vi "Main.vi"(11 "Module Admin":refnum<class "Delacor_lib_QMH_Module Admin.lvclass">) -> ()   [LabVIEW 2020, in "Panter Dashboard.lvlib"]
doc: "This template is based off of the Queued Message Handler design pattern and the Queued Message Handler project template that ships with LabVIEW.\n\nThe main difference is that the queue is private to this module and communication between modules is performed via Broadcast and Request events.\n\nRequest events are wrapped in public API methods and are handled in the Event Handling Loop (EHL) of this VI. Any module can register for Broadcast events sent by this module. The EHL generates messages based on user interface actions.\n\nThe Message Handling Loop (MHL) processes messages generated by the EHL, or by other messages. The messages are string values, so new messages can be added easily to the Message Cases case structure in the MHL. Each message cluster can also provide an optional value for Message Data, which is a variant that can be converted to whatever message-specific data is required.\n_____\nBased on DQMH Project Template 6.1.0.94."
uses:
  Panter Dashboard.lvlib
  <vilib>/Delacor/Delacor QMH/Libraries/Module Admin_class/Delacor_lib_QMH_Module Admin.lvclass
  Search button.ctl
  Module type--enum.ctl
  Module Data--cluster.ctl
  Maps List and refs--cluster.ctl
  <vilib>/National Instruments/Tree Map/Tree Map Data.ctl
  DQMH Modules Info--cluster.ctl
  Stop Argument--cluster.ctl
  <vilib>/Delacor/Delacor QMH/Libraries/Message Queue_class/Delacor_lib_QMH_Message Queue.lvclass/Delacor_lib_QMH_Message Queue.ctl
  Scan DQMH Modules Argument--cluster.ctl
  Tree DQMH Selection Argument--cluster.ctl
  Open Module API Tester Argument--cluster.ctl
  Open Event Front Panel Argument--cluster.ctl
  Execute Default Event Request Argument--cluster.ctl
  DQMH Tools Menu--enum.ctl
  Stop Module Instance Argument--cluster.ctl
  <vilib>/Delacor/Delacor QMH/Libraries/Module Admin_class/Delacor_lib_QMH_Module Admin.lvclass/Delacor_lib_QMH_Module Admin.ctl
  <vilib>/Delacor/Delacor QMH/Libraries/Module Admin_class/Delacor_lib_QMH_Get External Launch.vi
  <vilib>/Delacor/Delacor QMH/Libraries/Message Queue_class/Delacor_lib_QMH_Enqueue Message (Single).vi
  <vilib>/National Instruments/Tree Map/API/List Roots.vi
  <vilib>/National Instruments/Tree Map/Utility/Into Tree Control Items.vi
  <vilib>/Utility/error.llb/Error Cluster From Error Code.vi
  <vilib>/ErrorRing/Error Ring.xnode
  <vilib>/Delacor/Delacor QMH/Libraries/Message Queue_class/Delacor_lib_QMH_Message Queue.lvclass
  <vilib>/National Instruments/Tree Map/Tree Map.lvlib
panel:
  in  "Include Dependencies":bool
  in  "Scan Project For DQMH® Modules":T1
  in  "Modules Tree":string(tree) caption="Tree 2"
  out "Running?":bool
  out "Module type":T2
  out "Event Connector Pane":picture
  in  "Open Event FP":bool
  in  "Open API Tester":bool
  out "Module Description":string
  out "Event Description":string
  in  "Module ID":i32 caption="Numeric" format="Module ID : %d"
  in  "Show Diagram":bool
  in  "Hide Panel":bool
  in  "Show Panel":bool
  in  "Stop Instance":bool
  in  "Validate Module":bool
  in  "Rename Module":bool
  in  "Add Module":bool
  in  "Rename Event":bool
  in  "Convert Event":bool
  in  "Remove Event":bool
  in  "Add Event":bool
  out "Messages":string
  out "error out":errorcluster
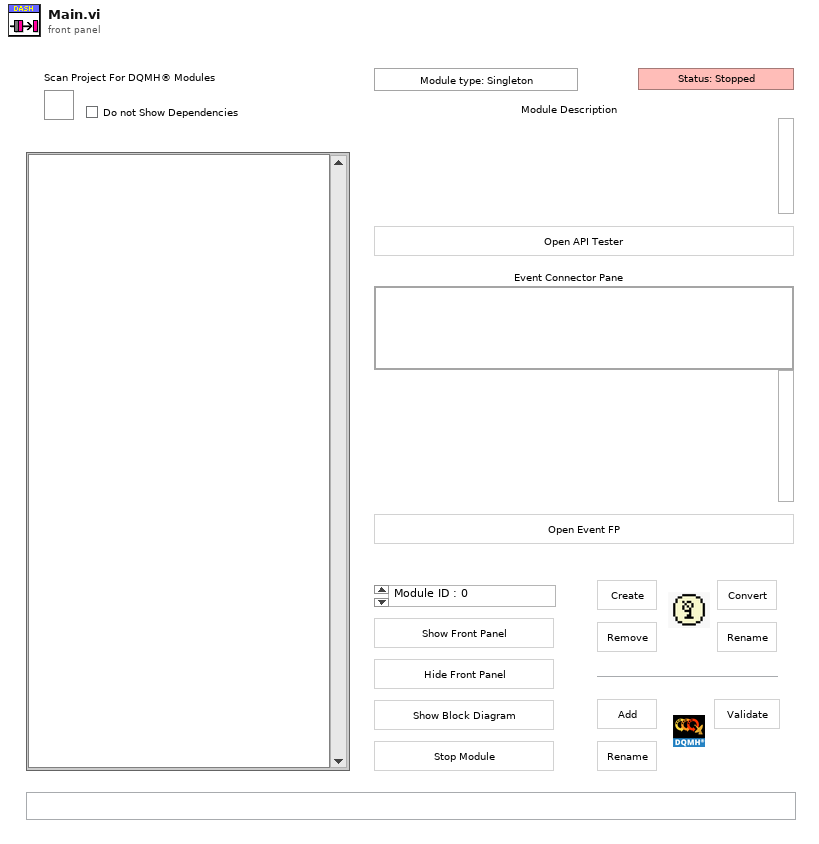
[diagram p1: front panel]
types:
  T1 = typedef "Panter Dashboard.lvlib/Search button.ctl" = bool
  T2 = typedef "Panter Dashboard.lvlib/Module type--enum.ctl" = enum16{"Module type: Singleton", "Module type: Cloneable"}
  T3 = typedef "Panter Dashboard.lvlib/Broadcast Events--cluster.ctl" = cluster{"Module Did Init":refnum<user-event>, "Status Updated":refnum<user-event>, "Error Reported":refnum<user-event>, "Module Did Stop":refnum<user-event>, "Update Module Execution Status":refnum<user-event>, "References Updated":refnum<user-event>}
  T4 = typedef "Panter Dashboard.lvlib/Request Events--cluster.ctl" = cluster{"Stop Module":refnum<user-event>, "Show Panel":refnum<user-event>, "Hide Panel":refnum<user-event>, "Get Module Execution Status":refnum<user-event>, "Show Diagram":refnum<user-event>, "Scan DQMH Modules":refnum<user-event>, "Tree DQMH Selection":refnum<user-event>, "Open Module API Tester":refnum<user-event>, "Open Event Front Panel":refnum<user-event>, "Execute Default Event Request":refnum<user-event>, "Stop Module Instance":refnum<user-event>}
  T5 = typedef "Panter Dashboard.lvlib/Module Data--cluster.ctl" = cluster{"DQMH Refs":cluster{"Event vi Ref":refnum<vi>, "DQMH Module Selected Ref":refnum<vi>}, "Status":string, "Maps":T6, "DQMH Modules Info":T8, "Module type":T2, "Module ID":i32}
  T6 = typedef "Panter Dashboard.lvlib/Maps List and refs--cluster.ctl" = cluster{"Tree Map":T7, "References Map":map{string, refnum<vi>}}
  T7 = typedef "Tree Map.lvlib/Tree Map Data.ctl" = map{string, cluster{"Child Paths Set":set{string}, "Name":string, "Data":string, "Attributes":map{string, string}}}
  T8 = typedef "Panter Dashboard.lvlib/DQMH Modules Info--cluster.ctl" = cluster{"DQMH Modules Refs":refnum<vi>[], "Modules List":string[], "Modules Descriptions":string[], "Modules Paths":path[], "Modules type":T2[]}
  T9 = enum32{"invalid lock state", "Not Locked", "Locked (No Password)", "Password-protected"}
  T10 = typedef "Panter Dashboard.lvlib/Stop Argument--cluster.ctl" = cluster{"Origin":string, "Exit via Stop Module Req?":bool, "Wait for Module to stop?":bool}
  T11 = typedef "Panter Dashboard.lvlib/Scan DQMH Modules Argument--cluster.ctl" = cluster{"Include Dependencies":bool}
  T12 = typedef "Panter Dashboard.lvlib/Tree DQMH Selection Argument--cluster.ctl" = cluster{"Tree DQMH Sel":string}
  T13 = typedef "Panter Dashboard.lvlib/Open Module API Tester Argument--cluster.ctl" = cluster{"Boolean":bool}
  T14 = typedef "Panter Dashboard.lvlib/Open Event Front Panel Argument--cluster.ctl" = cluster{"Boolean":bool}
  T15 = typedef "Panter Dashboard.lvlib/Execute Default Event Request Argument--cluster.ctl" = cluster{"Event Name":string}
  T16 = typedef "Panter Dashboard.lvlib/DQMH Tools Menu--enum.ctl" = enum16{"Create New DQMH Event", "Remove DQMH Event", "Convert DQMH Event", "Rename DQMH Event", "Add New DQMH Module", "Create RT Tester", "Rename DQMH Module", "Validate DQMH Module", "Create DQMH Module Template", "New DQMH  Unit Test"}
  T17 = typedef "Panter Dashboard.lvlib/Stop Module Instance Argument--cluster.ctl" = cluster{"Boolean":bool}
  T18 = enum32{"Invalid", "Standard", "Closed", "Hidden", "Minimized", "Maximized"}
  T19 = enum8{"Enabled", "Disabled", "Disabled and Grayed Out"}
  T20 = cluster{"Left Cell String":string, "Child Text":string[], "Child Tag":string, "Item Indent":i32, "Child Only?":bool, "Glyph Index":i32}[]
  T21 = typedef "Panter Dashboard.lvlib/Documentation--cluster.ctl" = cluster{"Module Description":string, "Event Description":string}
  T22 = cluster{"Vi out":refnum<vi>, "DQMH Lib":refnum<vi>}
  T23 = cluster{"Event vi Ref":refnum<vi>, "DQMH Module Selected Ref":refnum<vi>}
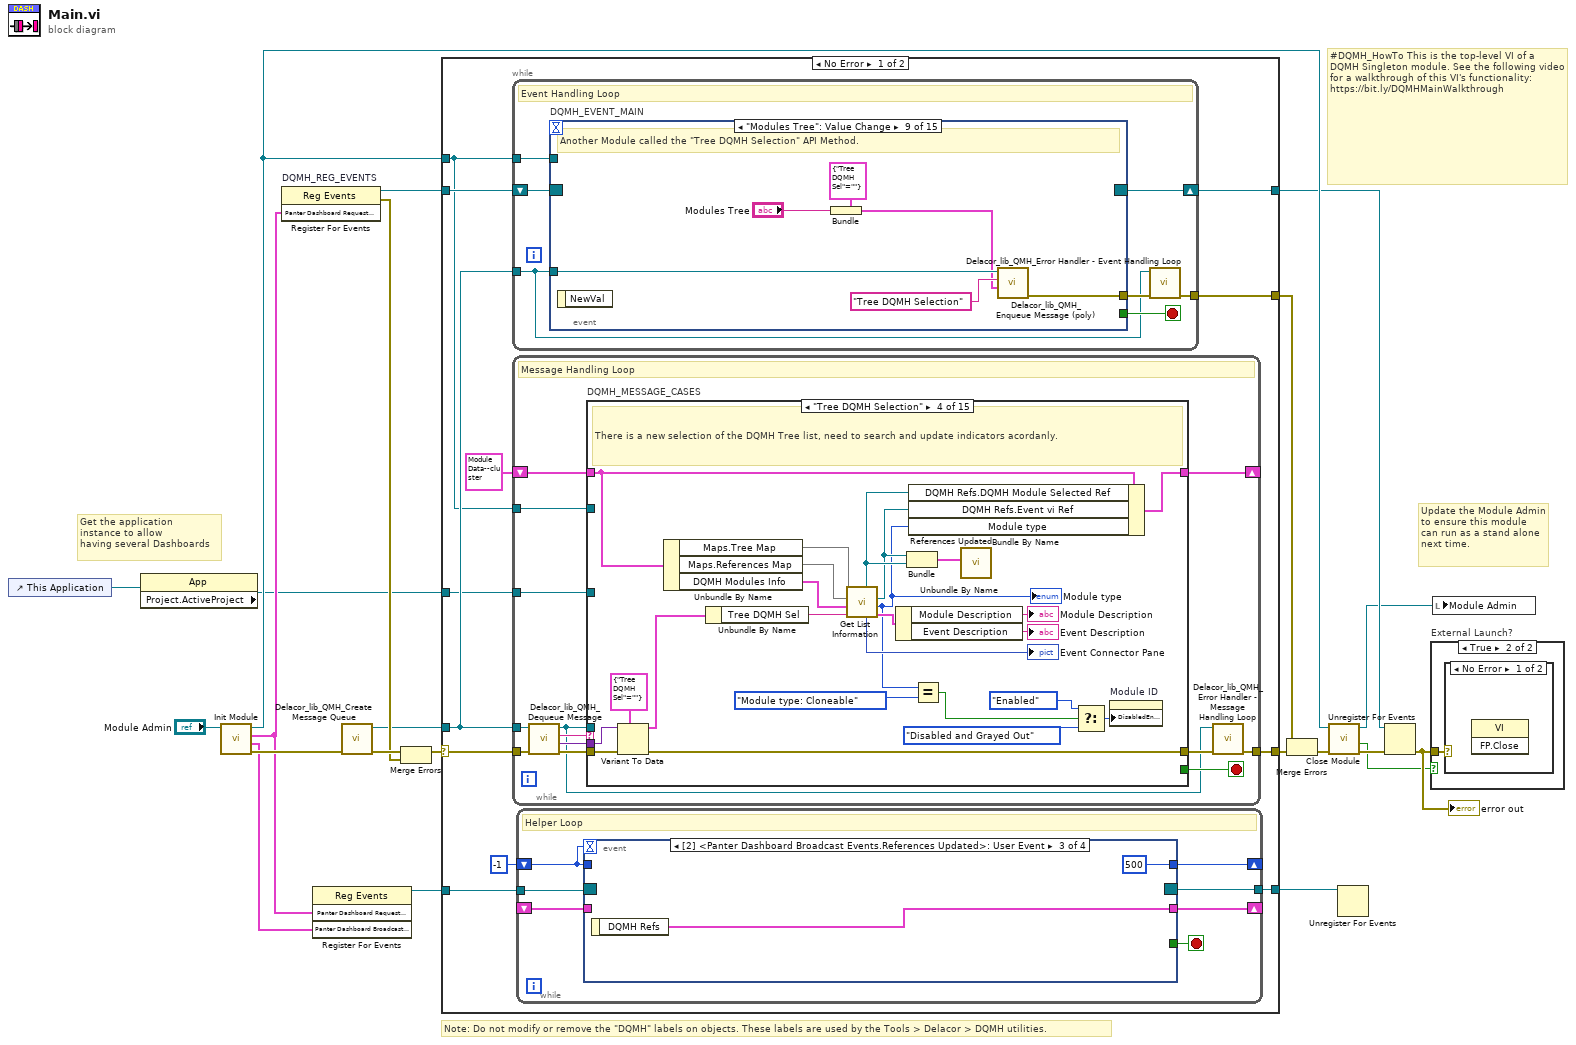
[diagram p0: block diagram]
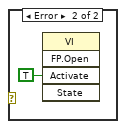
[diagram p3: hidden frame]
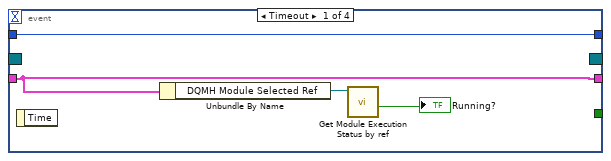
[diagram p4: hidden frame]
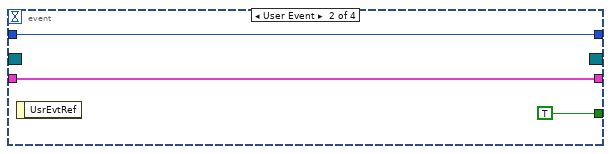
[diagram p5: hidden frame]
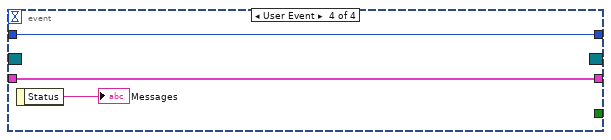
[diagram p6: hidden frame]
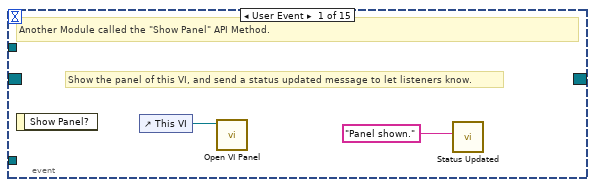
[diagram p7: hidden frame]
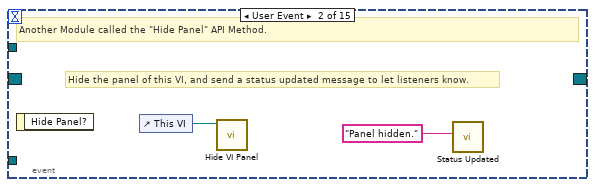
[diagram p8: hidden frame]
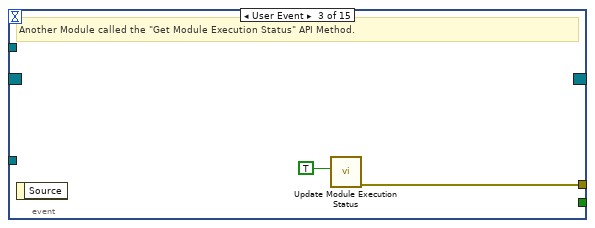
[diagram p9: hidden frame]
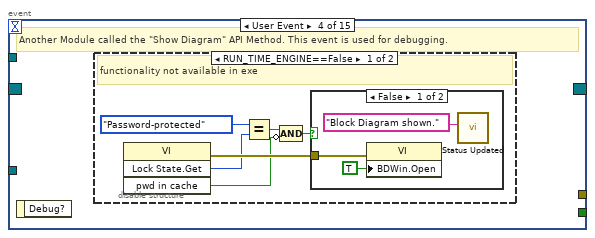
[diagram p10: hidden frame]
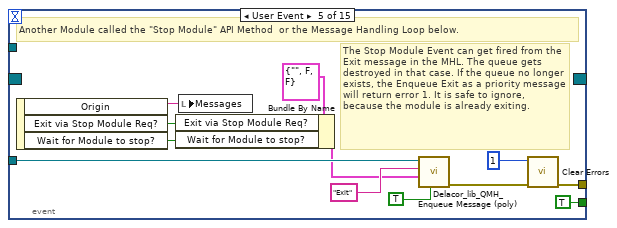
[diagram p13: hidden frame]
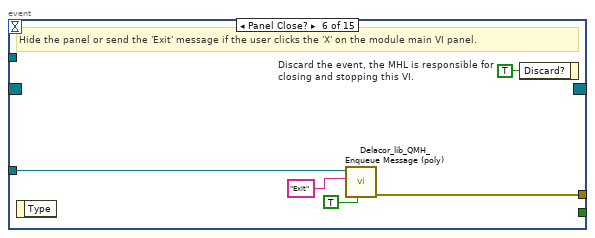
[diagram p14: hidden frame]
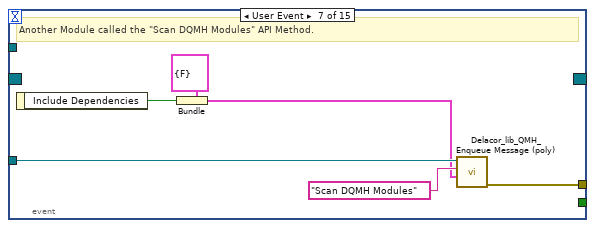
[diagram p15: hidden frame]
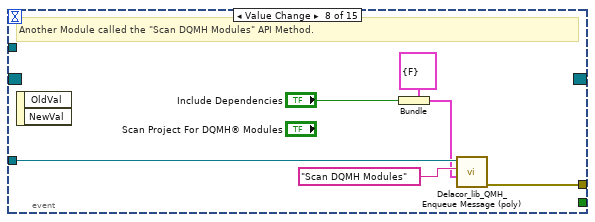
[diagram p16: hidden frame]
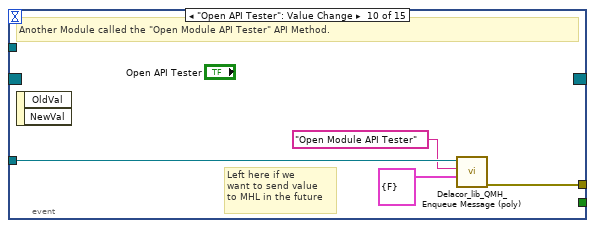
[diagram p17: hidden frame]
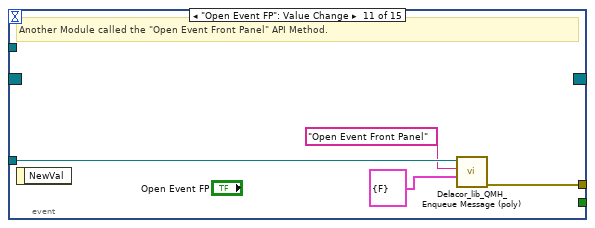
[diagram p18: hidden frame]
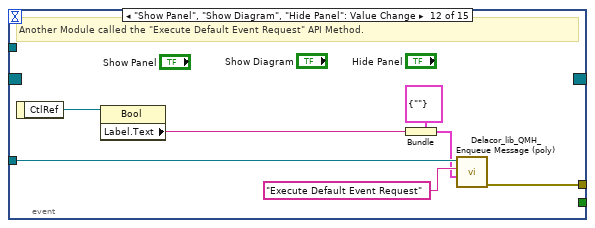
[diagram p19: hidden frame]
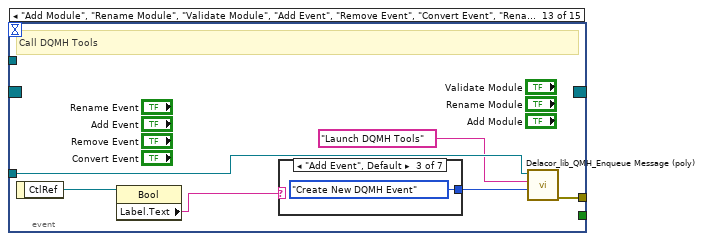
[diagram p20: hidden frame]
diagram:
  # "Get the application\ninstance to allow\nhaving several Dashboards"
  # "#DQMH_HowTo This is the top-level VI of a DQMH Singleton module. See the following video for a walkthrough of this VI's functionality: https://bit.ly/DQMHMainWalkthrough"
  # "Note: Do not modify or remove the \"DQMH\" labels on objects. These labels are used by the Tools > Delacor > DQMH utilities."
  # "Update the Module Admin to ensure this module can run as a stand alone next time."
  n1 = control-ref of="This Application"() -> (w2:refnum<vi>)
  n2 = property class="App"(reference=w2) -> ("Project.ActiveProject"=w1:refnum<vi>)  [unwired: 1 in, 2 out]
  n3 = call "Init Module.vi"("Singleton Module Admin in"="Module Admin") -> ("error out"=w21:errorcluster, "Panter Dashboard Broadcast Events"=w3:T3, "Panter Dashboard Request Events"=w4:T4, "Singleton Module Admin out"=w13:refnum<class "Delacor_lib_QMH_Module Admin.lvclass">)  [unwired: 7 in]
  n4 = register-events "DQMH_REG_EVENTS"(w4) -> (reference out=w11:refnum<event-registration>, error out=w14:errorcluster)  [unwired: 2 in]
  n5 = register-events(w4, w3) -> (reference out=w6:refnum<event-registration>)  [unwired: 2 in, 1 out]
  n6 = call <vilib>:"Delacor_lib_QMH_Create Message Queue.vi"("error in"=w21) -> ("error out"=w16:errorcluster, "Message Queue"=w10:refnum<class "Delacor_lib_QMH_Message Queue.lvclass">)  [unwired: 9 in]
  n7 = Merge Errors(w16, w14) -> (w15:errorcluster)
  n8 = case shown="No Error" w15 {
    selector: w15 -> [w32 w344]
    tunnel: [w34 w343] -> w22
    tunnel: [w31 w342] -> w12
    tunnel: w11 -> [w29 w342]
    tunnel: w10 -> [w28 w337]
    tunnel: [w33 _] -> w19
    tunnel: w13 -> [w27 w338]
    tunnel: w6 -> [w26 w336]
    tunnel: [w25 w336] -> w5
    tunnel: w1 -> [w23 _]
    frame No Error {
      n9 = while {
        tunnel: w28 -> [w54]
        shift-right: [w57] -> w31
        shift-left: w29 -> [w58]
        tunnel: [w59] -> w33
        tunnel: w27 -> [w55]
        stop <- w56 stop-if-true
        # "Event Handling Loop"
        n10 = event "DQMH_EVENT_MAIN" shown="[8] \"Modules Tree\": Value Change" {
          selector: w58 -> [_ _ _ _ _ _ _ _ _ _ _ _ _ _ _]
          dyn-events: [_ _ _ _ _ _ _ _ _ _ _ _ _ _ _] -> w57
          timeout: _ -> [_ _ _ _ _ _ _ _ _ _ _ _ _ _ _]
          tunnel: [_ _ _ _ TRUE ("Discard?") _ _ _ _ _ _ _ _ _ _] -> w56
          tunnel: w54 -> [_ _ _ _ w83 w90 w97 w103 w109 w113 w117 w124 w130 w141 w145]
          tunnel: [_ _ w66 _ w86 w92 w98 w104 w110 w114 w118 w125 w131 w142 w146] -> w60
          tunnel: w55 -> [_ _ _ _ _ _ _ _ _ _ _ _ _ _ _]
          event User Event {
            # "Show the panel of this VI, and send a status updated message to let listeners know."
            # "Another Module called the \"Show Panel\" API Method."
            n11 = event-data() -> ()  [unwired: 1 in, 1 out]
            n12 = control-ref of="This VI"() -> (w62:refnum<vi>)
            n13 = call "Open VI Panel.vi"("VI"=w62) -> ()  [unwired: 10 in, 1 out]
            n14 = call "Status Updated.vi"("Status"="Panel shown." ("format string")) -> ()  [unwired: 10 in, 1 out]
          }
          event User Event {
            # "Hide the panel of this VI, and send a status updated message to let listeners know."
            # "Another Module called the \"Hide Panel\" API Method."
            n15 = event-data() -> ()  [unwired: 1 in, 1 out]
            n16 = control-ref of="This VI"() -> (w64:refnum<vi>)
            n17 = call "Hide VI Panel.vi"("VI"=w64) -> ()  [unwired: 10 in, 1 out]
            n18 = call "Status Updated.vi"("Status"="Panel hidden." ("format string")) -> ()  [unwired: 10 in, 1 out]
          }
          event User Event {
            # "Another Module called the \"Get Module Execution Status\" API Method."
            n19 = event-data() -> ()  [unwired: 1 in, 1 out]
            n20 = call "Update Module Execution Status.vi"("Running?"=TRUE) -> ("error out"=w66:errorcluster)  [unwired: 10 in]
          }
          event User Event {
            # "Another Module called the \"Show Diagram\" API Method. This event is used for debugging."
            n21 = event-data() -> ()  [unwired: 1 in, 1 out]
            n22 = disable-structure shown="RUN_TIME_ENGINE==False" {
              frame condition #0 (active) {
                # "functionality not available in exe"
                n23 = invoke class="VI" method="Lock State.Get"() -> (error out=w72:errorcluster, "Get Lock State"=w71:T9, "pwd in cache"=w68:bool)  [unwired: 4 in, 1 out]
                n24 = Equal?(x=T9."Password-protected", y=w71) -> (x = y?=w69:bool)
                n25 = Compound Arithmetic op=AND(w69, invert w68) -> (w67:bool)
                n26 = case shown="False" w67 {
                  tunnel: w72 -> [w75 _]
                  frame False {
                    n27 = property class="VI"(error in=w75, "BDWin.Open"=TRUE ("Block Diagram Window:Open")) -> ()  [unwired: 1 in, 2 out]
                    n28 = call "Status Updated.vi"("Status"="Block Diagram shown." ("format string")) -> ()  [unwired: 10 in, 1 out]
                  }
                  frame True {
                    # "Password-protected VI, and the password is not in the cache. Do not show the diagram."
                  }
                }
              }
              frame condition #1 {
              }
            }
          }
          event User Event {
            # "The Stop Module Event can get fired from the Exit message in the MHL. The queue gets destroyed in that case. If the queue no longer exists, the Enqueue Exit as a priority message will return error 1. It is safe to ignore, because the module is already exiting."
            # "Another Module called the \"Stop Module\" API Method  or the Message Handling Loop below."
            n29 = event-data() -> ("Origin"=w82:string, "Exit via Stop Module Req?"=w78:bool, "Wait for Module to stop?"=w77:bool)  [unwired: 1 in]
            n30 = Bundle By Name(cluster=T10 {"Origin"="", "Exit via Stop Module Req?"=FALSE, "Wait for Module to stop?"=FALSE} ("Stop Argument"), "Exit via Stop Module Req?"=w78, "Wait for Module to stop?"=w77) -> (w76:T10)
            n31 = local write "Messages"(w82) -> ()
            n32 = call-poly <vilib>:"Delacor_lib_QMH_Enqueue Message (poly).vi"("Priority Message? (F)"=TRUE, "Message Data"=w76, "Message"="Exit", "Message Queue in"=w83) -> ("error out"=w87:errorcluster)  [unwired: 6 in, 1 out]
            n33 = call <vilib>:"Clear Errors.vi"("error in (no error)"=w87, "specific error code to clear (0: all)"=1) -> ("error out"=w86:errorcluster)  [unwired: 4 in, 1 out]
          }
          event Panel Close? {
            w91 = TRUE  # Discard the event, the MHL is responsible for closing and stopping this VI.
            # "Hide the panel or send the 'Exit' message if the user clicks the 'X' on the module main VI panel."
            n34 = event-data() -> ()  [unwired: 1 in, 1 out]
            n35 = call-poly <vilib>:"Delacor_lib_QMH_Enqueue Message (poly).vi"("Priority Message? (F)"=TRUE, "Message"="Exit", "Message Queue in"=w90) -> ("error out"=w92:errorcluster)  [unwired: 7 in, 1 out]
            n36 = event-data("Discard?"=w91) -> ()  [unwired: 1 in, 1 out]
          }
          event User Event {
            # "Another Module called the \"Scan DQMH Modules\" API Method."
            n37 = event-data() -> ("Include Dependencies"=w93:bool)  [unwired: 1 in]
            n38 = Bundle(cluster=T11 {"Include Dependencies"=FALSE} ("Scan DQMH Modules Argument"), "Include Dependencies"=w93) -> (w94:T11)
            n39 = call-poly <vilib>:"Delacor_lib_QMH_Enqueue Message (poly).vi"("Message Data"=w94, "Message"="Scan DQMH Modules", "Message Queue in"=w97) -> ("error out"=w98:errorcluster)  [unwired: 7 in, 1 out]
          }
          event Value Change {
            # "Another Module called the \"Scan DQMH Modules\" API Method."
            n40 = event-data() -> ()  [unwired: 1 in, 2 out]
            n41 = Bundle(cluster=T11 {"Include Dependencies"=FALSE} ("Scan DQMH Modules Argument"), "Include Dependencies"="Include Dependencies") -> (w100:T11)
            n42 = call-poly <vilib>:"Delacor_lib_QMH_Enqueue Message (poly).vi"("Message Data"=w100, "Message"="Scan DQMH Modules", "Message Queue in"=w103) -> ("error out"=w104:errorcluster)  [unwired: 7 in, 1 out]
          }
          event "Modules Tree": Value Change {
            # "Another Module called the \"Tree DQMH Selection\" API Method."
            n43 = event-data() -> ()  [unwired: 1 in, 1 out]
            n44 = Bundle(cluster=T12 {"Tree DQMH Sel"=""} ("Tree DQMH Selection Argument"), "Tree DQMH Sel"="Modules Tree") -> (w106:T12)
            n45 = call-poly <vilib>:"Delacor_lib_QMH_Enqueue Message (poly).vi"("Message Data"=w106, "Message"="Tree DQMH Selection", "Message Queue in"=w109) -> ("error out"=w110:errorcluster)  [unwired: 7 in, 1 out]
          }
          event "Open API Tester": Value Change {
            # "Left here if we\nwant to send value\nto MHL in the future"
            # "Another Module called the \"Open Module API Tester\" API Method."
            n46 = event-data() -> ()  [unwired: 1 in, 2 out]
            n47 = call-poly <vilib>:"Delacor_lib_QMH_Enqueue Message (poly).vi"("Message Data"=T13 {"Boolean"=FALSE} ("Open Module API Tester Argument"), "Message"="Open Module API Tester", "Message Queue in"=w113) -> ("error out"=w114:errorcluster)  [unwired: 7 in, 1 out]
          }
          event "Open Event FP": Value Change {
            # "Another Module called the \"Open Event Front Panel\" API Method."
            n48 = event-data() -> ()  [unwired: 1 in, 1 out]
            n49 = call-poly <vilib>:"Delacor_lib_QMH_Enqueue Message (poly).vi"("Message Data"=T14 {"Boolean"=FALSE} ("Open Event Front Panel Argument"), "Message"="Open Event Front Panel", "Message Queue in"=w117) -> ("error out"=w118:errorcluster)  [unwired: 7 in, 1 out]
          }
          event "Show Panel", "Show Diagram", "Hide Panel": Value Change {
            # "Another Module called the \"Execute Default Event Request\" API Method."
            n50 = event-data() -> ("CtlRef"=w120:refnum<vi>)  [unwired: 1 in]
            n51 = property class="Bool"(reference=w120) -> ("Label.Text"=w119:string)  [unwired: 1 in, 2 out]
            n52 = Bundle(cluster=T15 {"Event Name"=""} ("Execute Default Event Request Argument"), "Event Name"=w119) -> (w121:T15)
            n53 = call-poly <vilib>:"Delacor_lib_QMH_Enqueue Message (poly).vi"("Message Data"=w121, "Message"="Execute Default Event Request", "Message Queue in"=w124) -> ("error out"=w125:errorcluster)  [unwired: 7 in, 1 out]
          }
          event "Add Module", "Rename Module", "Validate Module", "Add Event", "Remove Event", "Convert Event", "Rename Event": Value Change {
            # "Call DQMH Tools"
            n54 = event-data() -> ("CtlRef"=w127:refnum<vi>)  [unwired: 1 in]
            n55 = property class="Bool"(reference=w127) -> ("Label.Text"=w126:string)  [unwired: 1 in, 2 out]
            n56 = case shown="\"Add Event\", Default" w126 {
              tunnel: [DQMH_Tools_Menu--enum."Remove DQMH Event" ("DQMH Tools") DQMH_Tools_Menu--enum."Rename DQMH Event" ("DQMH Tools") DQMH_Tools_Menu--enum."Create New DQMH Event" ("DQMH Tools") DQMH_Tools_Menu--enum."Convert DQMH Event" ("DQMH Tools") DQMH_Tools_Menu--enum."Add New DQMH Module" ("DQMH Tools") DQMH_Tools_Menu--enum."Validate DQMH Module" ("DQMH Tools") DQMH_Tools_Menu--enum."Rename DQMH Module" ("DQMH Tools")] -> w128
              frame "Remove Event" {
              }
              frame "Rename Event" {
              }
              frame "Add Event", Default {
              }
              frame "Convert Event" {
              }
              frame "Add Module" {
              }
              frame "Validate Module" {
              }
              frame "Rename Module" {
              }
            }
            n57 = call-poly <vilib>:"Delacor_lib_QMH_Enqueue Message (poly).vi"("Message Data"=w128, "Message"="Launch DQMH Tools", "Message Queue in"=w130) -> ("error out"=w131:errorcluster)  [unwired: 7 in, 1 out]
          }
          event "Stop Instance": Value Change {
            # "Another Module called the \"Stop Module Instance\" API Method."
            n58 = event-data() -> ()  [unwired: 1 in, 1 out]
            n59 = call-poly <vilib>:"Delacor_lib_QMH_Enqueue Message (poly).vi"("Message Data"=T17 {"Boolean"=FALSE} ("Stop Module Instance Argument"), "Message"="Stop Module Instance", "Message Queue in"=w141) -> ("error out"=w142:errorcluster)  [unwired: 7 in, 1 out]
          }
          event "Module ID": Value Change {
            # "Module ID has value change"
            n60 = event-data() -> ()  [unwired: 1 in, 1 out]
            n61 = call-poly <vilib>:"Delacor_lib_QMH_Enqueue Message (poly).vi"("Message Data"="Module ID", "Message"="Module ID Update", "Message Queue in"=w145) -> ("error out"=w146:errorcluster)  [unwired: 7 in, 1 out]
          }
        }
        n62 = call-dynamic "Delacor_lib_QMH_Error Handler - Event Handling Loop.vi"("error in"=w60, "Message Queue in"=w54) -> ("dup error in"=w59:errorcluster)  [unwired: 8 in, 1 out]
      }
      n63 = while {
        tunnel: w28 -> [w150]
        shift-right: [w154] -> _
        shift-left: T5 {"DQMH Refs"={"Event vi Ref"=refnum, "DQMH Module Selected Ref"=refnum}, "Status"="", "Maps"={"Tree Map"={}, "References Map"={}}, "DQMH Modules Info"={"DQMH Modules Refs"=[], "Modules List"=[], "Modules Descriptions"=[], "Modules Paths"=[], "Modules type"=[]}, "Module type"=enum."Module type: Singleton", "Module ID"=0} ("Data Cluster") -> [w155]
        tunnel: w32 -> [w158]
        tunnel: [w156] -> w34
        tunnel: w27 -> [w148]
        tunnel: w23 -> [w147]
        stop <- w153 stop-if-true
        # "Message Handling Loop"
        n64 = call-dynamic "Delacor_lib_QMH_Dequeue Message.vi"("error in"=w158, "Message Queue in"=w150) -> ("error out"=w157:errorcluster, "Message Data"=w151:variant, "Message"=w152:string, "Message Queue out"=w149:refnum<class "Delacor_lib_QMH_Message Queue.lvclass">)  [unwired: 6 in]
        n65 = case "DQMH_MESSAGE_CASES" shown="\"Tree DQMH Selection\"" w152 {
          selector: w152 -> [_ _ _ _ _ _ _ _ _ _ _ _ _ _ w323]
          tunnel: w149 -> [_ _ _ _ _ _ _ _ _ _ _ _ w292 w315 _]
          tunnel: w157 -> [w180 w184 w202 w226 w233 w242 w253 w266 w277 w284 w287 w289 w299 w321 w325]
          tunnel: [w178 w184 w200 w225 w232 w241 w252 w264 w275 w283 w286 w289 w295 w318 w326] -> w159
          tunnel: w155 -> [w169 w183 w185 w220 w230 w238 w247 w259 w271 w282 w285 w288 w294 w307 w324]
          tunnel: [w168 w183 w195 w212 w230 w238 w247 w259 w271 w280 w285 w288 w294 w307 w324] -> w154
          tunnel: [_ _ _ _ _ _ _ _ _ _ _ _ _ w314 _] -> w153
          tunnel: w151 -> [_ _ w198 w224 w229 w240 w251 w262 w273 w281 _ _ w293 w313 _]
          tunnel: w148 -> [w170 _ _ _ _ _ _ _ _ _ _ _ w291 w308 _]
          tunnel: w147 -> [w163 _ w187 _ _ _ _ _ _ _ _ _ _ _ _]
          frame "Initialize" {
            w164 = "Panther Dash " ("Initial Message")
            # "Initialize - Any operation that needs to be done before the module can receive messages. Synchronize Caller Events.vi will inform Start Module.vi that the module has launched and is ready to receive messages. Module Did Init.vi will broadcast that the module initialized."
            n66 = call "Synchronize Caller Events.vi"("error in (no error)"=w180, "Singleton Module Admin in"=w170) -> ("error out"=w179:errorcluster, "Singleton Module Admin out"=w165:refnum<class "Delacor_lib_QMH_Module Admin.lvclass">)  [unwired: 8 in]
            n67 = property class="Project"(reference=w163) -> ("Name"=w162:string)  [unwired: 1 in, 2 out]
            n68 = property class="Module Admin"(reference=w165) -> ("Accessors:External Launch"=w174:bool)  [unwired: 1 in, 2 out]
            n69 = invoke on="Modules Tree" class="Tree (strict)" method="Edit Tree Items.Delete"() -> ()  [unwired: 5 in, 5 out]
            n70 = Select(t=T18."Hidden" ("State"), s=w174, f=T18."Standard" ("State")) -> (s? t:f=w171:T18)
            n71 = Format Into String(format string="Panther Dasboard for DQMH® : %s", w162) -> (resulting string=w161:string, error out=w177:errorcluster)  [unwired: 2 in]
            n72 = property class="VI"(error in=w177, "Front Panel.Title"=w161) -> (reference out=w176:refnum<vi>, error out=w182:errorcluster)  [unwired: 1 in]
            n73 = call "Module Name--constant.vi"() -> ("Module Name"=w166:string)  [unwired: 11 in]
            n74 = invoke class="VI" method="FP.Open"(reference=w176, error in=w182, "State"=w171) -> (reference out=w175:refnum<vi>, error out=w181:errorcluster)  [unwired: 2 in, 3 out]
            n75 = Bundle By Name(cluster=w169, "Status"=w164) -> (w168:T5)
            n76 = local write "Messages"(w164) -> ()
            n77 = call "Module Did Init.vi"("error in (no error)"=w179, "Initialized?"=TRUE, "Origin"=w166) -> ("error out"=w178:errorcluster)  [unwired: 8 in]
            n78 = invoke class="VI" method="FP.Center"(reference=w175, error in=w181) -> ()  [unwired: 1 in, 3 out]
          }
          frame "---Module Specific---" {
            # "Separator -- The following cases handle messages specific to this Module."
          }
          frame "Scan DQMH Modules" {
            # "Scan DQMH Modules in the project and fill 2 maps one with the Vi References and the another one with the list of DQMH modules on the project"
            n79 = Variant To Data(error in=w202, type=T11 {"Include Dependencies"=FALSE} ("Scan DQMH Modules Argument"), Variant=w198) -> (data=w196:T11, error out=w201:errorcluster)
            n80 = Unbundle By Name(w196) -> ("Include Dependencies"=w186:bool)
            n81 = local write "Include Dependencies"(w186) -> ()
            n82 = call "Get Panther Dash Library.vi"() -> ("Library out"=w193:refnum<vi>)  [unwired: 11 in]
            n83 = call "Scan DQMH Modules and create Maps.vi"("Panther Dash DQMH Lib"=w193, "Include Dependencies"=w186, "Project"=w187) -> ("error out"=w199:errorcluster, "Tree Map out"=w188:T7, "map ref out"=w189:map{string, refnum<vi>}, "DQMH Modules Info"=w194:T8)  [unwired: 5 in]
            n84 = control-ref of="Modules Tree"() -> (w190:refnum<vi>)
            n85 = Bundle By Name(cluster=w185, "DQMH Modules Info"=w194, "Maps.References Map"=w189, "Maps.Tree Map"=w188) -> (w195:T5)
            n86 = call <vilib>:"Tree Map to Tree Control Items.vi"("Tree Map In"=w188) -> ("Tree Control Items"=w191:T20)  [unwired: 10 in]
            n87 = call "Draw Tree.vi"("Tree Control Items"=w191, "TreeControl in"=w190) -> ()  [unwired: 9 in, 1 out]
            n88 = Merge Errors(w201, w199) -> (w200:errorcluster)
            n89 = call "Status Updated.vi"("Status"="Scanning DQMH Modules") -> ()  [unwired: 10 in, 1 out]
          }
          frame "Tree DQMH Selection" {
            # "There is a new selection of the DQMH Tree list, need to search and update indicators acordanly."
            n90 = Variant To Data(error in=w226, type=T12 {"Tree DQMH Sel"=""} ("Tree DQMH Selection Argument"), Variant=w224) -> (data=w222:T12, error out=w225:errorcluster)
            n91 = Unbundle By Name(w220) -> ("Maps.Tree Map"=w219:T7, "Maps.References Map"=w218:map{string, refnum<vi>}, "DQMH Modules Info"=w217:T8)
            n92 = Unbundle By Name(w222) -> ("Tree DQMH Sel"=w221:string)
            n93 = call "Get List Information.vi"("List Selection"=w221, "DQMH Modules Info"=w217, "References Map"=w218, "Tree Map"=w219) -> ("Documentation"=w215:T21, "Module Type"=w205:T2, "Vi out"=w210:refnum<vi>, "VI Connector Pane"=→"Event Connector Pane":picture, "DQMH Lib"=w211:refnum<vi>)  [unwired: 2 in, 1 out]
            "Module type" <- w205
            n94 = Unbundle By Name(w215) -> ("Module Description"=→"Module Description":string, "Event Description"=→"Event Description":string)
            n95 = Bundle("Vi out"=w210, "DQMH Lib"=w211) -> (w209:T22)  [unwired: 1 in]
            n96 = Bundle By Name(cluster=w220, "DQMH Refs.DQMH Module Selected Ref"=w211, "DQMH Refs.Event vi Ref"=w210, "Module type"=w205) -> (w212:T5)
            n97 = Equal?(x=w205, y=Module_type--enum."Module type: Cloneable") -> (x = y?=w204:bool)
            n98 = call "References Updated.vi"("DQMH Refs"=w209) -> ()  [unwired: 10 in, 1 out]
            n99 = Select(t=T19."Enabled" ("Disabled"), s=w204, f=T19."Disabled and Grayed Out") -> (s? t:f=w207:T19)
            n100 = property on="Module ID" class="DigNum (strict)"("DisabledEnum"=w207) -> ()  [unwired: 2 in, 2 out]
          }
          frame "Launch DQMH Tools" {
            # "Launch DQMH Tools"
            n101 = Variant To Data(error in=w233, type=DQMH_Tools_Menu--enum."Create New DQMH Event" ("DQMH Tools"), Variant=w229) -> (data=w227:T16, error out=w231:errorcluster)
            n102 = call "Launch DQMH Tools by menu.vi"("error in"=w231, "DQMH Tools"=w227) -> ("error out"=w232:errorcluster)  [unwired: 9 in]
          }
          frame "Open Module API Tester" {
            # "Open the API Tester from the selected DQMH Module"
            n103 = Variant To Data(error in=w242, type=T13 {"Boolean"=FALSE} ("Open Module API Tester Argument"), Variant=w240) -> ()  [unwired: 2 out]
            n104 = Unbundle By Name(w238) -> ("DQMH Refs.DQMH Module Selected Ref"=w236:refnum<vi>)
            n105 = property class="Library"(reference=w236) -> ("Name"=w235:string)  [unwired: 1 in, 2 out]
            n106 = call "Open API Tester.vi"("DQMH Library Ref"=w236) -> ("error out"=w241:errorcluster)  [unwired: 10 in]
            n107 = Format Into String(format string="Open: %s  API Tester " ("Status"), w235) -> (resulting string=w234:string)  [unwired: 2 in, 1 out]
            n108 = call "Status Updated.vi"("Status"=w234) -> ()  [unwired: 10 in, 1 out]
          }
          frame "Open Event Front Panel" {
            # "Open the Front Panel from the selected Event from the tree"
            n109 = Variant To Data(error in=w253, type=T14 {"Boolean"=FALSE} ("Open Event Front Panel Argument"), Variant=w251) -> ()  [unwired: 2 out]
            n110 = Unbundle By Name(w247) -> ("DQMH Refs.Event vi Ref"=w246:refnum<vi>)
            n111 = invoke class="VI" method="FP.Open"(reference=w246, "Activate"=TRUE ("Wait Until Done"), "State"=T18."Standard") -> (error out=w252:errorcluster)  [unwired: 2 in, 4 out]
            n112 = property class="VI"(reference=w246) -> ("Name"=w245:string)  [unwired: 1 in, 2 out]
            n113 = Format Into String(format string="Front Panel : %s Opened", w245) -> (resulting string=w244:string)  [unwired: 2 in, 1 out]
            n114 = call "Status Updated.vi"("Status"=w244) -> ()  [unwired: 10 in, 1 out]
          }
          frame "Execute Default Event Request" {
            # "Execute Default Event"
            n115 = Unbundle By Name(w259) -> ("Maps.References Map"=w258:map{string, refnum<vi>}, "DQMH Refs.DQMH Module Selected Ref"=w257:refnum<vi>, "Module type"=w255:T2, "Module ID"=w254:i32)
            n116 = Variant To Data(error in=w266, type=T15 {"Event Name"=""} ("Execute Default Event Request Argument"), Variant=w262) -> (data=w260:T15, error out=w265:errorcluster)
            n117 = Unbundle By Name(w260) -> ("Event Name"=w256:string)
            n118 = call "Execute default event by ID.vi"("Event Name"=w256, "Module ID"=w254, "Module type"=w255, "Module Lib"=w257, "References Map"=w258) -> ("error out"=w263:errorcluster)  [unwired: 6 in]
            n119 = Merge Errors(w265, w263) -> (w264:errorcluster)
          }
          frame "Stop Module Instance" {
            # "Execute the Stop Module Request, when Cloneable type this Request uses the Module ID"
            n120 = Variant To Data(error in=w277, type=T17 {"Boolean"=FALSE} ("Stop Module Instance Argument"), Variant=w273) -> (error out=w276:errorcluster)  [unwired: 1 out]
            n121 = Unbundle By Name(w271) -> ("Maps.References Map"=w270:map{string, refnum<vi>}, "DQMH Refs.DQMH Module Selected Ref"=w269:refnum<vi>, "Module type"=w268:T2, "Module ID"=w267:i32)
            n122 = call "Stop DQMH Module.vi"("Module ID"=w267, "Module type"=w268, "Module Lib"=w269, "References Map"=w270) -> ("error out"=w274:errorcluster)  [unwired: 7 in]
            n123 = Merge Errors(w276, w274) -> (w275:errorcluster)
          }
          frame "Module ID Update" {
            # "Module ID Control has value change"
            n124 = Variant To Data(error in=w284, type=0 ("Module ID"), Variant=w281) -> (data=w279:i32, error out=w283:errorcluster)
            n125 = Bundle By Name(cluster=w282, "Module ID"=w279) -> (w280:T5)
          }
          frame "---Copy This Frame---" {
            # "Duplicate this frame when creating new messages.  Change this comment in the duplicated frame to describe this message."
            n126 = Merge Errors(w287) -> (w286:errorcluster)
          }
          frame "---Exit and Error Handling---" {
            # "Separator - The following cases handle errors and exit messages."
          }
          frame "Error" {
            # "#CodeRecommended - If you ever change the name of this \"Error\" message, you'll need to update the name in the Check Loop Error.vi as well."
            # "#CodeRecommended - If the module is running in standalone mode (External Launch = FALSE), this code will pop up an error dialog and call the 'Exit' message if an error occurs. Add more fine-grained error handling here."
            # "Error - Check the error message data and respond accordingly. This message is sent by the \"Error Handler\" VIs at the end of each loop in this application."
            n127 = property class="Module Admin"(reference=w291) -> ("Accessors:External Launch"=w290:bool)  [unwired: 1 in, 2 out]
            n128 = Variant To Data(error in=w299, type=errorcluster {"status"=FALSE, "code"=0, "source"=""} ("error constant"), Variant=w293) -> (data=w300:errorcluster, error out=w297:errorcluster)
            n129 = call "Error Reported.vi"("Error"=w300) -> ()  [unwired: 10 in, 1 out]
            n130 = case shown="False" w290 {
              tunnel: [w305 _] -> w296
              tunnel: w292 -> [w303 _]
              tunnel: w300 -> [w304 _]
              frame False {
                # "If the module is running standalone, then pop up an error dialog and call the \"Exit\" message."
                n131 = call <vilib>:"Simple Error Handler.vi"("error in (no error)"=w304) -> ()  [unwired: 4 in, 5 out]
                n132 = call-poly <vilib>:"Delacor_lib_QMH_Enqueue Message (poly).vi"("Priority Message? (F)"=TRUE, "Message"="Exit", "Message Queue in"=w303) -> ("error out"=w305:errorcluster)  [unwired: 7 in, 1 out]
              }
              frame True {
                # "If the module was launched externally, calling the Error Reported broadcast VI is the only action performed by the \"Error\" message. The module's caller can then process the error appropriately."
              }
            }
            n133 = Merge Errors(w297, w296) -> (w295:errorcluster)
            n134 = local write "error out"(w295) -> ()
          }
          frame "Exit" {
            w312 = 91  # 91: not all Exit messages will have an argument
            w314 = TRUE  # Stop the VI
            # "Release the message queue reference"
            # "#CodeNeeded - Add any required cleanup code here"
            # "Exit - Exit the application."
            n135 = Variant To Data(error in=w321, type=T10 {"Origin"="", "Exit via Stop Module Req?"=FALSE, "Wait for Module to stop?"=FALSE} ("Stop Argument"), Variant=w313) -> (data=w310:T10, error out=w317:errorcluster)
            n136 = call <vilib>:"Clear Errors.vi"("error in (no error)"=w317, "specific error code to clear (0: all)"=w312) -> ("error out"=w320:errorcluster)  [unwired: 4 in, 1 out]
            n137 = control-ref of="This VI"() -> (w309:refnum<vi>)
            n138 = call-dynamic "Delacor_lib_QMH_Release Message Queue.vi"("error in"=w320, "Message Queue"=w315) -> ("error out"=w319:errorcluster)  [unwired: 9 in]
            n139 = call "Handle Exit.vi"("Stop Argument"=w310, "Admin in"=w308, "VI reference"=w309) -> ("error out"=w316:errorcluster)  [unwired: 7 in, 1 out]
            n140 = Unbundle By Name(w307) -> ("Maps.References Map"=w306:map{string, refnum<vi>})
            n141 = Merge Errors(w319, w316) -> (w318:errorcluster)
            n142 = call "Close vi references.vi"("map"=w306) -> ()  [unwired: 10 in, 1 out]
          }
          frame Default {
            # "'Default' case only runs if there is a message that isn't defined in any of the other cases.  Output a programming error."
            n143 = call "Module Name--constant.vi"() -> ("Module Name"=w322:string)  [unwired: 11 in]
            n144 = xnode "Error Ring"("parameter 0"=w323, "parameter 1"=w322) -> ("error out"=w327:errorcluster)
            n145 = Merge Errors(w325, w327) -> (w326:errorcluster)
          }
        }
        n146 = call-dynamic "Delacor_lib_QMH_Error Handler - Message Handling Loop.vi"("error in"=w159, "Message Queue in"=w149) -> ("dup error in"=w156:errorcluster)  [unwired: 8 in, 1 out]
      }
      n147 = while {
        tunnel: w26 -> [w41]
        tunnel: [w40] -> w25
        shift-right: [w38] -> _
        shift-left: -1 -> [w37]
        shift-right: [w36] -> _
        shift-left: _ -> [w35]
        stop <- w39 stop-if-true
        # "Helper Loop"
        n148 = event shown="[2] <Panter Dashboard Broadcast Events.References Updated>: User Event" {
          selector: w41 -> [_ _ _ _]
          dyn-events: [_ _ _ _] -> w40
          timeout: w37 -> [_ _ _ _]
          tunnel: [_ TRUE _ _] -> w39
          tunnel: [w44 w47 w50 w52] -> w36
          tunnel: [w45 w46 500 w51] -> w38
          tunnel: w37 -> [w45 w46 _ w51]
          tunnel: w35 -> [w44 w47 _ w52]
          event Timeout {
            n149 = event-data() -> ()  [unwired: 1 in, 1 out]
            n150 = Unbundle By Name(w44) -> ("DQMH Module Selected Ref"=w43:refnum<vi>)
            n151 = call "Get Module Execution Status by ref.vi"("Library"=w43) -> ("Running?"=→"Running?":bool)  [unwired: 8 in, 2 out]
          }
          event User Event {
            n152 = event-data() -> ()  [unwired: 1 in, 1 out]
          }
          event User Event {
            n153 = event-data() -> ("DQMH Refs"=w50:T23)  [unwired: 1 in]
          }
          event User Event {
            n154 = event-data() -> ("Status"=→"Messages":string)  [unwired: 1 in]
          }
        }
      }
    }
    frame Error {
      # "Synchronize Caller Events.vi will inform Start Module.vi that the module has launched and will let the code calling Start Module.vi register for broadcasts and would permit the caller receive the broadcast that an error occurred at launch time."
      n155 = call-dynamic "Delacor_lib_QMH_Release Message Queue.vi"("error in"=w344, "Message Queue"=w337) -> ("error out"=w343:errorcluster)  [unwired: 9 in]
      n156 = call "Synchronize Caller Events.vi"("Singleton Module Admin in"=w338) -> ("error out"=w345:errorcluster)  [unwired: 9 in, 1 out]
      n157 = call "Module Name--constant.vi"() -> ("Module Name"=w341:string)  [unwired: 11 in]
      n158 = Format Into String(format string="An error occurred during initialization. %s is no longer running.", w341) -> (resulting string=w339:string)  [unwired: 2 in, 1 out]
      n159 = Merge Errors(w343, w345) -> (w346:errorcluster)
      n160 = call "Error Reported.vi"("Additional Information"=w339, "Error"=w346) -> ()  [unwired: 9 in, 1 out]
    }
  }
  n161 = Merge Errors(w19, w22) -> (w18:errorcluster)
  n162 = call "Close Module.vi"("error in (no error)"=w18, "Module Admin in"=w13) -> ("error out"=w20:errorcluster, "External Launch"=w7:bool, "Module Admin out"=w8:refnum<class "Delacor_lib_QMH_Module Admin.lvclass">)  [unwired: 7 in]
  n163 = Unregister For Events(event registration refnum=w5) -> ()  [unwired: 1 in, 1 out]
  n164 = Unregister For Events(event registration refnum=w12, error in=w20) -> (error out=w17:errorcluster)
  "error out" <- w17
  n165 = case "External Launch?" shown="True" w7 {
    tunnel: w17 -> [_ w347]
    frame False {
    }
    frame True {
      n166 = case shown="No Error" w347 {
        frame No Error {
          n167 = invoke class="VI" method="FP.Close"() -> ()  [unwired: 3 in, 3 out]
        }
        frame Error {
          n168 = invoke class="VI" method="FP.Open"("Activate"=TRUE ("Activate?")) -> ()  [unwired: 4 in, 5 out]
        }
      }
    }
  }
  n169 = local write "Module Admin"(w8) -> ()
